vi "UV-VIS GetVSSpeed.vi"(4 "error in (no error)":errorcluster, 5 "index":i32, 7 "Control in":refnum<class "CCD_camera.lvclass">) -> (0 "error out":errorcluster, 1 "DLL error code":u32, 2 "speed":sgl format="%.2f", 3 "Control out":refnum<class "CCD_camera.lvclass">)   [LabVIEW 2020, in "CCD_camera.lvclass"]
doc: "As your AndorMCD[tm] system maybe capable of operating at more than one vertical shift speed this function will return the actual speeds available. The value returned is in microseconds per pixel shift.\n\n<B>Parameters:</B>\nindex - speed required\n Valid values: 0 to GetNumberVSSpeeds()-1\nspeed - speed in microseconds per pixel shift\n\n<B>Error codes:</B>\nDRV_SUCCESS - Speed returned.\nDRV_NOT_INITIALIZED - System not initialized.\nDRV_ACQUIRING - Acquisition in progress.\nDRV_P1INVALID - Invalid index."
uses:
  CCD_camera.lvclass
  C:/dev/TRANCON/Classes/Detector/Detector.lvclass
  Detector.lvclass/Detector.ctl
  Detector.lvclass
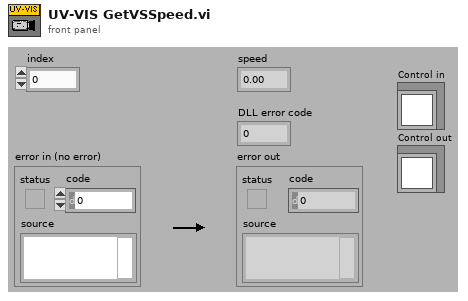
[diagram p1: front panel]
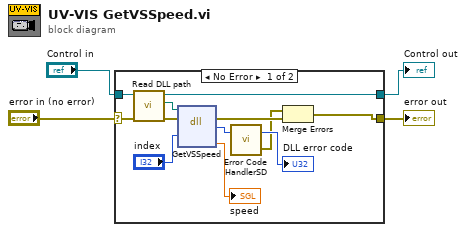
[diagram p0: block diagram]
diagram:
  n1 = case shown="No Error" "error in (no error)" {
    selector: "error in (no error)" -> [w11 w18]
    tunnel: [w6 w18] -> w3
    tunnel: [w5 w17] -> w2
    tunnel: "Control in" -> [w12 w17]
    frame No Error {
      n2 = call "Read DLL path.vi"("error in (no error)"=w11, "Detector in"=w12) -> ("error out"=w10:errorcluster, "DLL path"=w9:path, "Detector out"=w5:refnum<class "CCD_camera.lvclass">)  [unwired: 7 in]
      n3 = dll-call lib="S:/TRANCON/DLL/Atmcd32d.dll" fn="GetVSSpeed"(path in=w9, error in=w10, "index"="index") -> (error out=w8:errorcluster, "return type"=w16:u32, "speed"=→"speed":sgl)  [unwired: 3 in, 1 out]
      n4 = call "Error Code HandlerSD.vi"("DLL error code"=w16) -> ("error out"=w7:errorcluster, "dup DLL error code"=→"DLL error code":u32)  [unwired: 1 in]
      n5 = Merge Errors(w7, w8) -> (w6:errorcluster)
    }
    frame Error {
    }
  }
  "error out" <- w3
  "Control out" <- w2
